vi "Determine Frequency.vi"(6 "Sample Rate":i32, 7 "Signal (in)":dbl[](array[numeric]) format="%.2f") -> (3 "Fundamental frequency":dbl format="%.2f")   [LabVIEW 2013]
uses:
  <vilib>/measure/maspectr.llb/FFT Power Spectrum and PSD for 1 Chan.vi
  <vilib>/measure/NI_MAPro.lvlib
panel:
  out "power spectrum":cluster{"f0":dbl, "df":dbl, "magnitude":dbl[]}(graph)
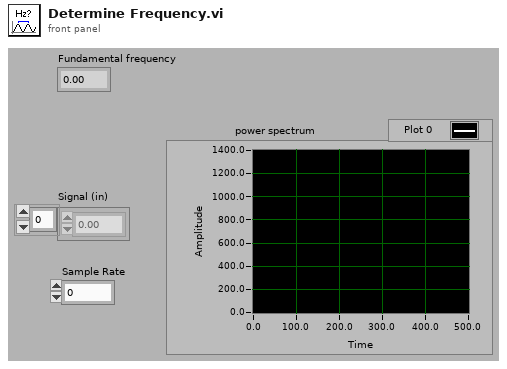
[diagram p1: front panel]
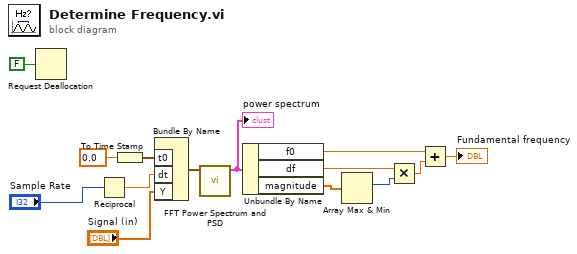
[diagram p0: block diagram]
diagram:
  n1 = Request Deallocation(FALSE ("flag")) -> ()
  n2 = Reciprocal(x="Sample Rate") -> (1/x=w12:dbl)
  n3 = To Time Stamp(1:0.0 ("t0")) -> (0:w2:timestamp)
  n4 = Bundle By Name("t0"=w2, "dt"=w12, "Y"="Signal (in)") -> (w10:waveform(dbl))  [unwired: 1 in]
  n5 = call-poly <vilib>:"FFT Power Spectrum and PSD.vi"("time signal"=w10) -> ("Power Spectrum / PSD"=w9:cluster{"f0":dbl, "df":dbl, "magnitude":dbl[]})  [unwired: 7 in, 3 out]
  "power spectrum" <- w9
  n6 = Unbundle By Name(w9) -> ("f0"=w4:dbl, "df"=w6:dbl, "magnitude"=w8:dbl[])
  n7 = Array Max & Min(array=w8) -> (max index (indices)=w7:i32)  [unwired: 3 out]
  n8 = Multiply(x=w6, y=w7) -> (x*y=w5:dbl)
  n9 = Add(x=w4, y=w5) -> (x+y=→"Fundamental frequency":dbl)
